vi "ProcessCalibrationData2.vi"(5 "Sensor Type":string, 7 "connection ID":refnum<k5>, 10 "Fiducial 2":dbl[][](array[numeric]) format="%#_8g", 11 "Fiducial 1":dbl[][](array[numeric]) format="%#_8g") -> (2 "Avg Length":dbl format="%0.2f")   [LabVIEW 2018]
uses:
  <vilib>/Analysis/baseanly.llb/Mean (DBL).vi
  <vilib>/Utility/file.llb/Write Delimited Spreadsheet (DBL).vi
  <vilib>/Analysis/NI_AALBase.lvlib
panel:
  out "error out 2":errorcluster
  out "error out":errorcluster
  # "Here a table of the co-ordinates for each interation of finding the fiducial can be found. Useful for debugging."
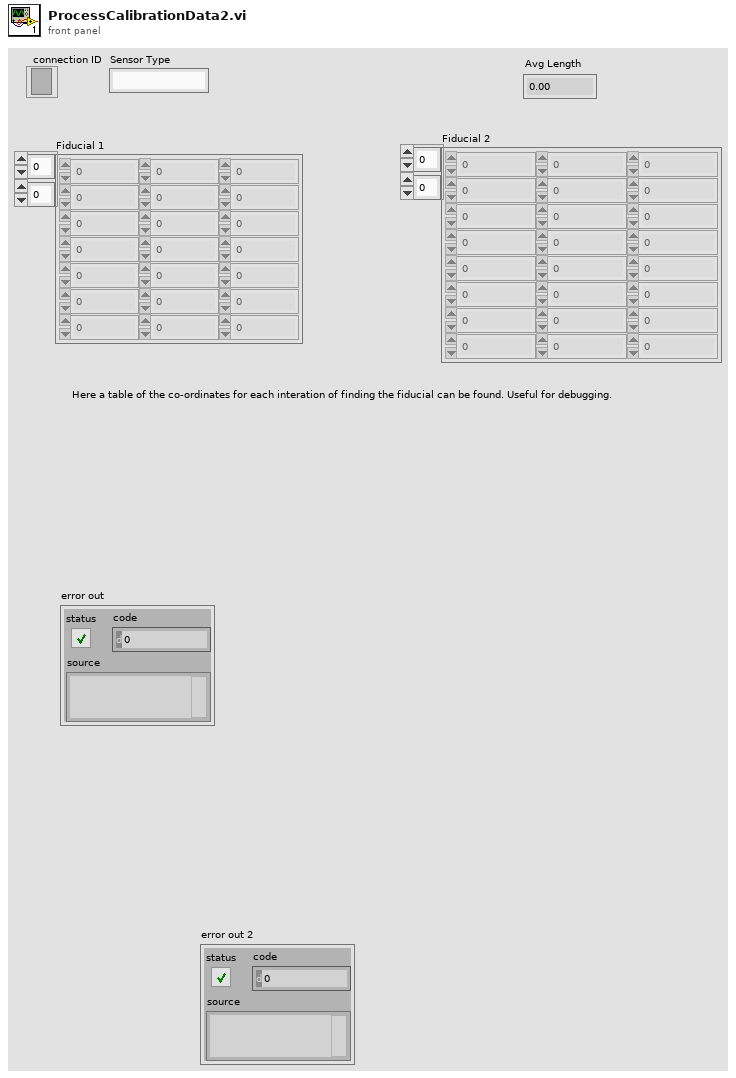
[diagram p1: front panel]
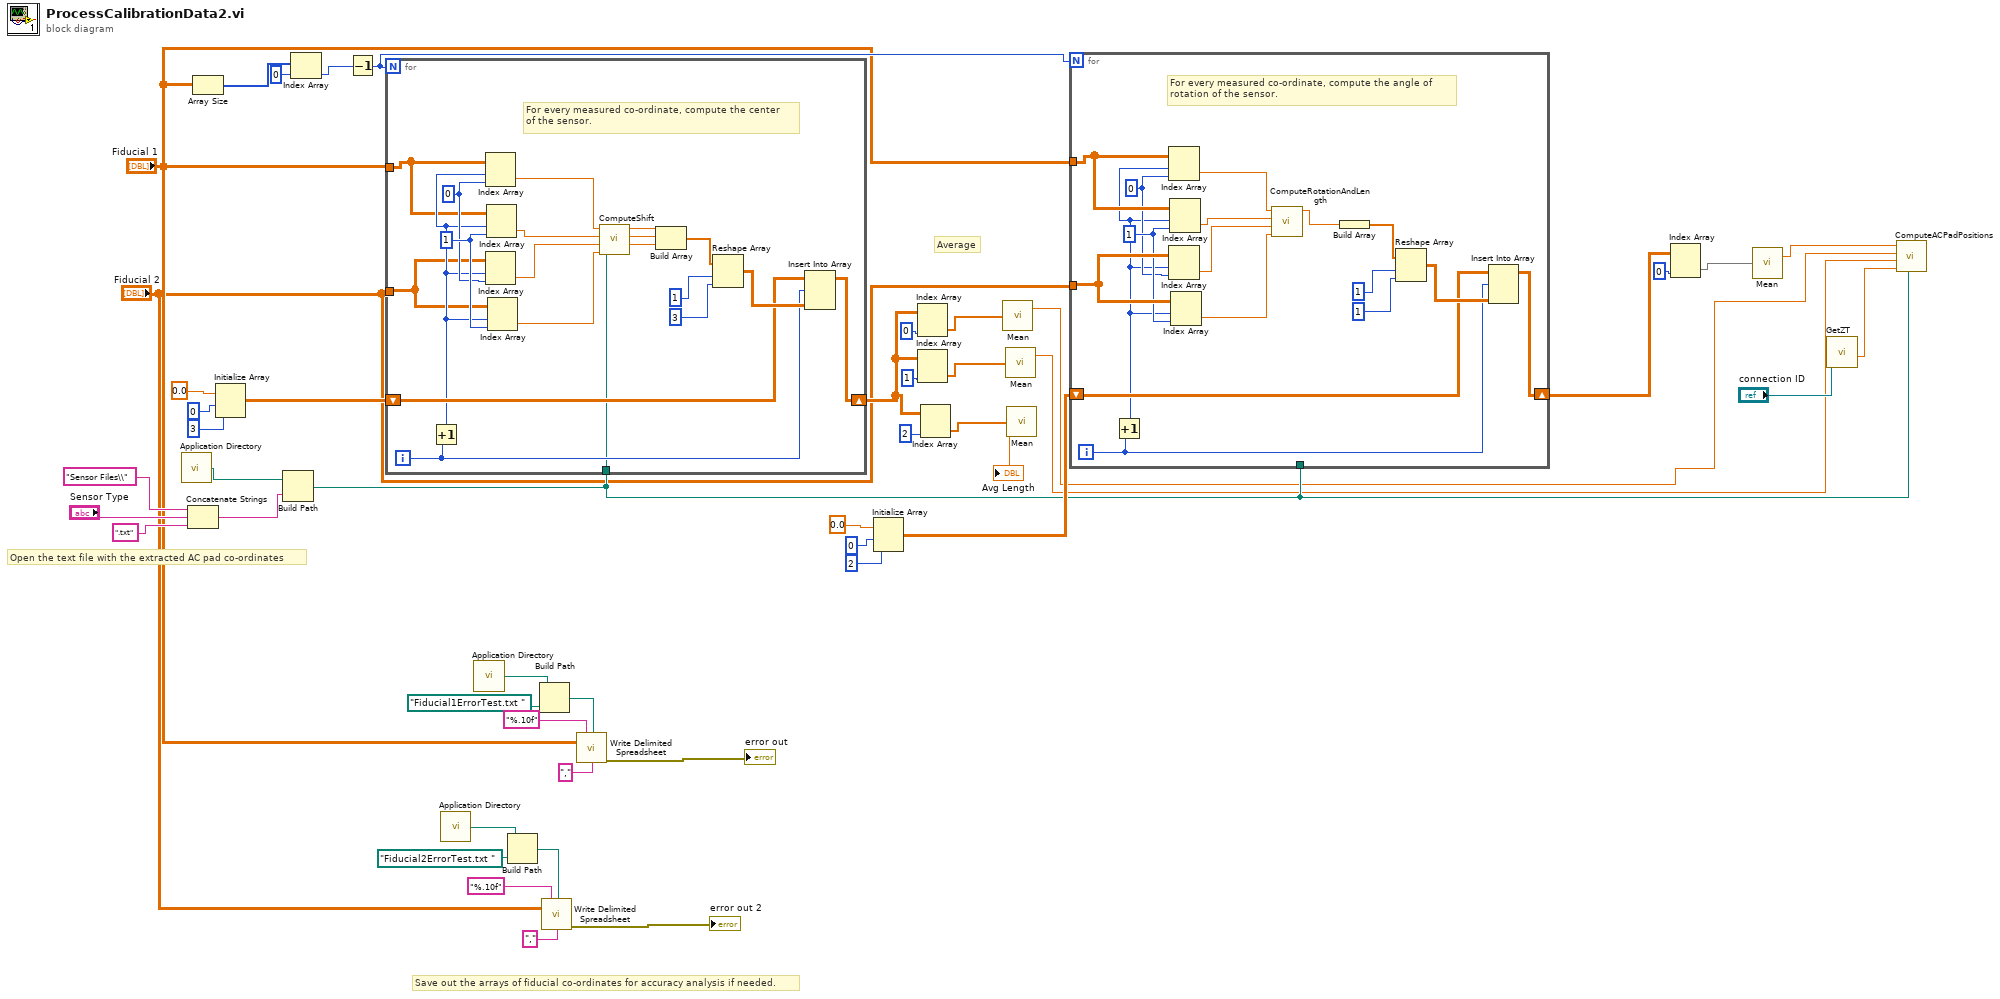
[diagram p0: block diagram]
diagram:
  # "Average"
  # "Save out the arrays of fiducial co-ordinates for accuracy analysis if needed."
  # "Open the text file with the extracted AC pad co-ordinates"
  n1 = call <vilib>:"Application Directory.vi"() -> ("Application Directory"=w34:path)
  n2 = Concatenate Strings("Sensor Files\\" ("string"), "Sensor Type", ".txt" ("string")) -> (w35:string)
  n3 = Array Size(array="Fiducial 1") -> (size(s)=w45:i32[])
  n4 = Initialize Array(0.0 ("element"), 0 ("dimension size"), 3 ("dimension size")) -> (w43:dbl[][])
  n5 = Build Path(base path=w34, name or relative path=w35) -> (appended path=w23:path)
  n6 = Index Array(array=w45, index=0) -> (element=w39:i32)
  n7 = Decrement(x=w39) -> (x-1=w24:i32)
  n8 = for {
    N: w24 -> [_]
    tunnel: "Fiducial 1" -> [w58]
    tunnel: "Fiducial 2" -> [w57]
    shift-right: [w62] -> w18
    shift-left: w43 -> [w61]
    tunnel: w23 -> [w56]
    i -> [w63]
    w68 = 1 ("disabled index (col)")
    w67 = 0 ("disabled index (col)")
    # "For every measured co-ordinate, compute the center\nof the sensor."
    n9 = Increment(x=w63) -> (x+1=w59:i32)
    n10 = Index Array(array=w58, index (row)=w59, index (col)=w67) -> (element=w52:dbl)
    n11 = Index Array(array=w57, index (row)=w59, index (col)=w67) -> (element=w54:dbl)
    n12 = Index Array(array=w58, index (row)=w59, index (col)=w68) -> (element=w53:dbl)
    n13 = Index Array(array=w57, index (row)=w59, index (col)=w68) -> (element=w55:dbl)
    n14 = call "ComputeShift.vi"("X1"=w52, "Y1"=w53, "X2"=w54, "Y2"=w55, "Path"=w56) -> ("XShift"=w51:dbl, "YShift"=w50:dbl, "Length"=w49:dbl)  [unwired: 3 in]
    n15 = Build Array(w51, w50, w49) -> (w65:dbl[])
    n16 = Reshape Array(w65, 1 ("dimension size"), 3 ("dimension size")) -> (w66:dbl[][])
    n17 = Insert Into Array(array=w61, index (row)=w63, new element=w66) -> (w62:dbl[][])  [unwired: 1 in]
  }
  n18 = call <vilib>:"Application Directory.vi"() -> ("Application Directory"=w7:path)
  n19 = call <vilib>:"Application Directory.vi"() -> ("Application Directory"=w13:path)
  n20 = Build Path(base path=w7, name or relative path=path "Fiducial2ErrorTest.txt " ("file path (dialog if empty)")) -> (appended path=w6:path)
  n21 = Build Path(base path=w13, name or relative path=path "Fiducial1ErrorTest.txt " ("file path (dialog if empty)")) -> (appended path=w12:path)
  n22 = call-poly <vilib>:"Write Delimited Spreadsheet.vi"("file path (dialog if empty)"=w6, "format (%.3f)"="%.10f", "2D data"="Fiducial 2", "delimiter (\\t)"="," ("delimiter (\\t)")) -> ("error out"=→"error out 2":errorcluster)  [unwired: 10 in, 1 out]
  n23 = call-poly <vilib>:"Write Delimited Spreadsheet.vi"("file path (dialog if empty)"=w12, "format (%.3f)"="%.10f", "2D data"="Fiducial 1", "delimiter (\\t)"="," ("delimiter (\\t)")) -> ("error out"=→"error out":errorcluster)  [unwired: 10 in, 1 out]
  n24 = Initialize Array(0.0 ("element"), 0 ("dimension size"), 2 ("dimension size")) -> (w25:dbl[][])
  n25 = Index Array(array=w18, index (col)=0 ("disabled index (col)")) -> (element=w33:dbl[])  [unwired: 1 in]
  n26 = Index Array(array=w18, index (col)=1 ("disabled index (col)")) -> (element=w32:dbl[])  [unwired: 1 in]
  n27 = Index Array(array=w18, index (col)=2 ("disabled index (col)")) -> (element=w16:dbl[])  [unwired: 1 in]
  n28 = call-poly <vilib>:"Mean.vi"("X"=w33) -> ("mean"=w21:dbl)  [unwired: 1 out]
  n29 = call-poly <vilib>:"Mean.vi"("X"=w32) -> ("mean"=w20:dbl)  [unwired: 1 out]
  n30 = call-poly <vilib>:"Mean.vi"("X"=w16) -> ("mean"=→"Avg Length":dbl)  [unwired: 1 out]
  n31 = for {
    N: w24 -> [_]
    tunnel: "Fiducial 1" -> [w85]
    tunnel: "Fiducial 2" -> [w84]
    shift-right: [w77] -> w19
    shift-left: w25 -> [w76]
    tunnel: w23 -> [_]
    i -> [w78]
    w83 = 1 ("disabled index (col)")
    w82 = 0 ("disabled index (col)")
    # "For every measured co-ordinate, compute the angle of \nrotation of the sensor."
    n32 = Increment(x=w78) -> (x+1=w74:i32)
    n33 = Index Array(array=w85, index (row)=w74, index (col)=w82) -> (element=w73:dbl)
    n34 = Index Array(array=w84, index (row)=w74, index (col)=w82) -> (element=w71:dbl)
    n35 = Index Array(array=w85, index (row)=w74, index (col)=w83) -> (element=w72:dbl)
    n36 = Index Array(array=w84, index (row)=w74, index (col)=w83) -> (element=w70:dbl)
    n37 = call "ComputeRotationAndLength.vi"("Y2"=w70, "X2"=w71, "Y1"=w72, "X1"=w73) -> ("Theta (Rad)"=w69:dbl)  [unwired: 7 in]
    n38 = Build Array(w69) -> (w80:dbl[])
    n39 = Reshape Array(w80, 1 ("dimension size"), 1 ("dimension size")) -> (w81:dbl[][])
    n40 = Insert Into Array(array=w76, index (row)=w78, new element=w81) -> (w77:dbl[][])  [unwired: 1 in]
  }
  n41 = Index Array(array=w19, index (col)=0 ("disabled index (col)")) -> (element=w29:dbl[])  [unwired: 1 in]
  n42 = call-poly <vilib>:"Mean.vi"("X"=w29) -> ("mean"=w22:dbl)  [unwired: 1 out]
  n43 = call "GetZT.vi"("connection ID"="connection ID") -> ("Theta (rad)"=w41:dbl)  [unwired: 7 in, 3 out]
  n44 = call "ComputeACPadPositions.vi"("Theta Calibration"=w22, "X cp"=w21, "Y cp"=w20, "Stage Initial\nRotation"=w41, "Sensor Path"=w23) -> ()  [unwired: 6 in]
